vi "DDG64.VI"() -> ()   [LabVIEW 2010]
panel:
  in  "gating":bool
  out "Calculated Kinetic Cycle Time":sgl format="%.2f"
  in  "Frequency (Hz):":dbl format="%.2f"
  in  "Integrate on chip":bool
  in  "Fast insertion delay":bool
  in  "Gate step (nsecs)":i32 step=25
  in  "Pulse Width (nsecs)":i32=1000
  in  "Delay (nsecs)":i32 step=25
  in  "Output A Delay (nsecs)":i32 min=0 step=16
  in  "Gain (0-255)":i32 min=0 max=255
  in  "Kinetic Cycle Time":sgl format="%.2f"
  in  "Shut Down":bool
  in  "Start Acquisition":bool
  out "Graphical Results":i32[](graph)
  out "Return  from Get Acquired Data":u32
  out "Detector X Pixels":i32
  out "Return from GetStatus":u32
  out "Return from Start Acquisition":u32
  in  "Number of Kinetics":i32=5
  out "Return from CheckTimings Exposure":u32
  out "Calculated Exposure Value":sgl format="%.2f"
  in  "Exposure Time (secs)":sgl=0.05 format="%.2f"
  out "Return from Initialize":u32
  in  "Trigger":u32(ring) items=["Internal", "External"]
  # "Status"
  # "Acquisition Mode: Kinetics\nReadout Mode: Full Vertical Binning.  Only showing one track of data."
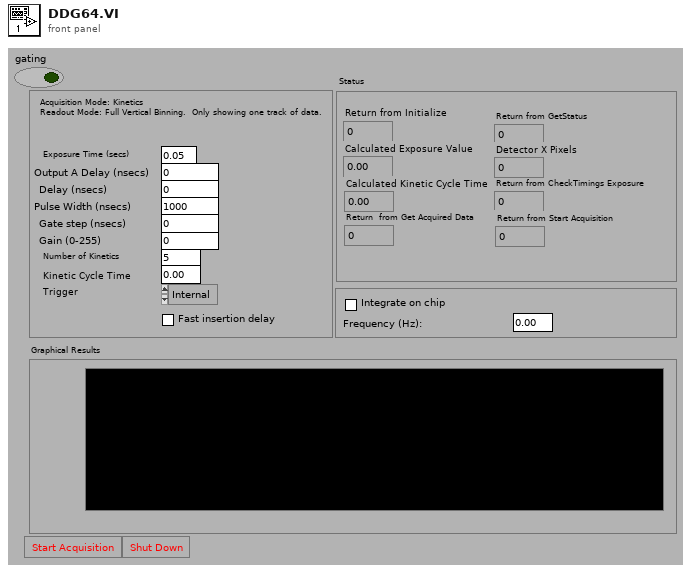
[diagram p1: front panel]
types:
  T1 = typedef "Error Code Enum typedef.ctl" = enum32{"N/A (0)", "DRV_ERROR_CODES", "DRV_SUCCESS", "DRV_VXDNOTINSTALLED", "DRV_ERROR_SCAN", "DRV_ERROR_CHECK_SUM", "DRV_ERROR_FILELOAD", "DRV_UNKNOWN_FUNC", "DRV_ERROR_VXD_INIT", "DRV_ERROR_ADDRESS", "DRV_ERROR_PAGELOCK", "DRV_ERROR_PAGEUNLOCK", "DRV_ERROR_BOARDTEST", "DRV_ERROR_ACK", "DRV_ERROR_UP_FIFO", "DRV_ERROR_PATTERN", "N/A (16)", "DRV_ACQUISITION_ERRORS", "DRV_ACQ_BUFFER", "DRV_ACQ_DOWNFIFO_FULL", "DRV_PROC_UNKONWN_INSTRUCTION", "DRV_ILLEGAL_OP_CODE", "DRV_KINETIC_TIME_NOT_MET", "DRV_ACCUM_TIME_NOT_MET", "DRV_NO_NEW_DATA", "N/A (25)", "DRV_SPOOLERROR", "N/A (27)", "N/A (28)", "N/A (29)", "N/A (30)", "N/A (31)", "N/A (32)", "DRV_TEMPERATURE_CODES", "DRV_TEMPERATURE_OFF", "DRV_TEMPERATURE_NOT_STABILIZED", "DRV_TEMPERATURE_STABILIZED", "DRV_TEMPERATURE_NOT_REACHED", "DRV_TEMPERATURE_OUT_RANGE", "DRV_TEMPERATURE_NOT_SUPPORTED", "DRV_TEMPERATURE_DRIFT", "N/A (41)", "N/A (42)", "N/A (43)", "N/A (44)", "N/A (45)", "N/A (46)", "N/A (47)", "N/A (48)", "DRV_GENERAL_ERRORS", "DRV_INVALID_AUX", "DRV_COF_NOTLOADED", "DRV_FPGAPROG", "DRV_FLEXERROR", "DRV_GPIBERROR", "N/A (55)", "N/A (56)", "N/A (57)", "N/A (58)", "N/A (59)", "N/A (60)", "N/A (61)", "N/A (62)", "N/A (63)", "DRV_DATATYPE", "DRV_DRIVER_ERRORS", "DRV_P1INVALID", "DRV_P2INVALID", "DRV_P3INVALID", "DRV_P4INVALID", "DRV_INIERROR", "DRV_COFERROR", "DRV_ACQUIRING", "DRV_IDLE", "DRV_TEMPCYCLE", "DRV_NOT_INITIALIZED", "DRV_P5INVALID", "DRV_P6INVALID", "DRV_INVALID_MODE", "DRV_INVALID_FILTER", "DRV_I2CERRORS", "DRV_I2CDEVNOTFOUND", "DRV_I2CTIMEOUT", "DRV_P7INVALID", "N/A (84)", "N/A (85)", "N/A (86)", "N/A (87)", "N/A (88)", "N/A (89)", "DRV_IOCERROR", "DRV_VRMVERSIONERROR"}
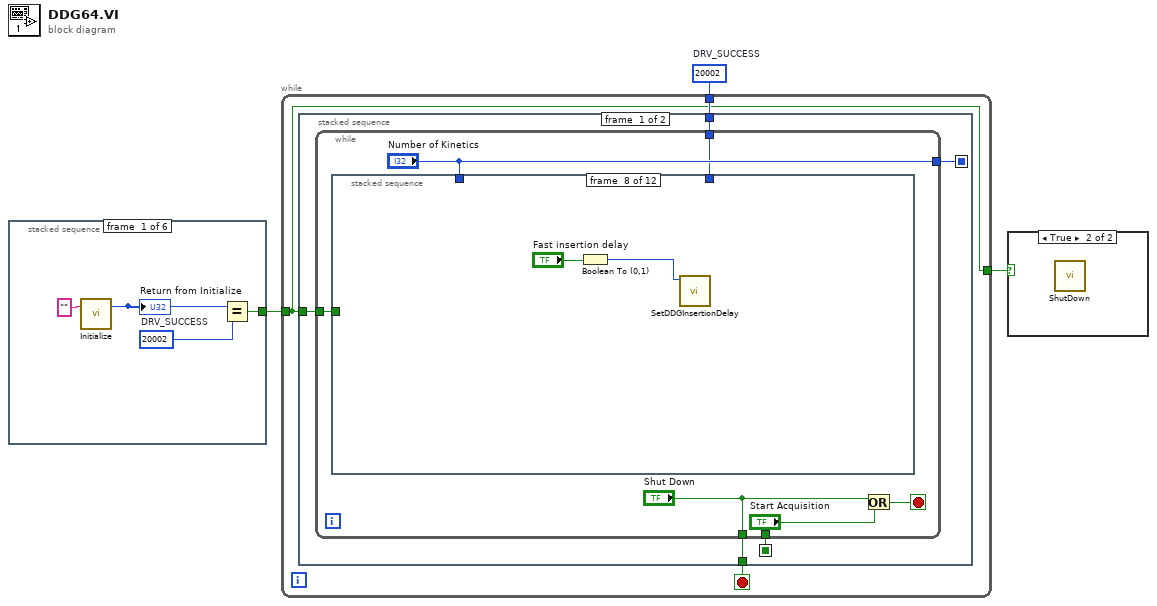
[diagram p0: block diagram]
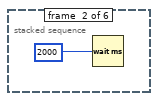
[diagram p2: hidden frame]
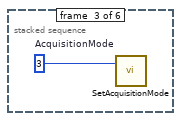
[diagram p3: hidden frame]
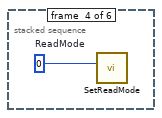
[diagram p4: hidden frame]
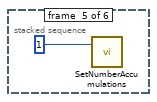
[diagram p5: hidden frame]
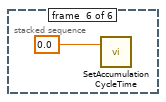
[diagram p6: hidden frame]
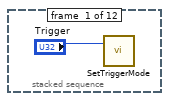
[diagram p8: hidden frame]
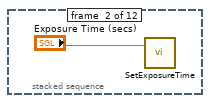
[diagram p9: hidden frame]
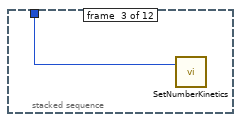
[diagram p10: hidden frame]
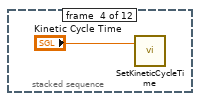
[diagram p11: hidden frame]
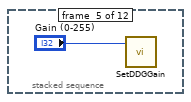
[diagram p12: hidden frame]
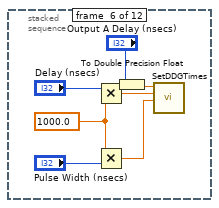
[diagram p13: hidden frame]
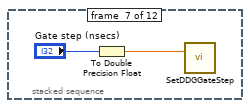
[diagram p14: hidden frame]
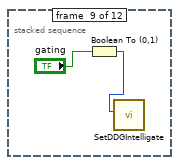
[diagram p15: hidden frame]
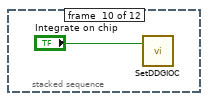
[diagram p16: hidden frame]
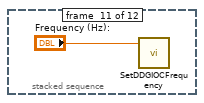
[diagram p17: hidden frame]
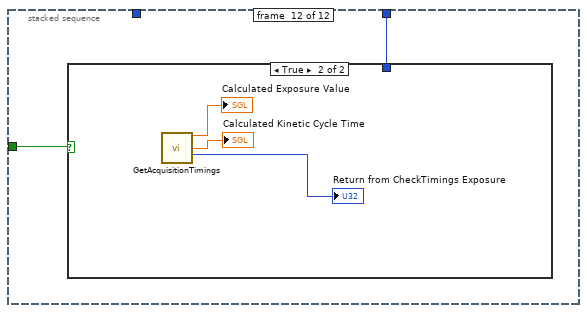
[diagram p18: hidden frame]
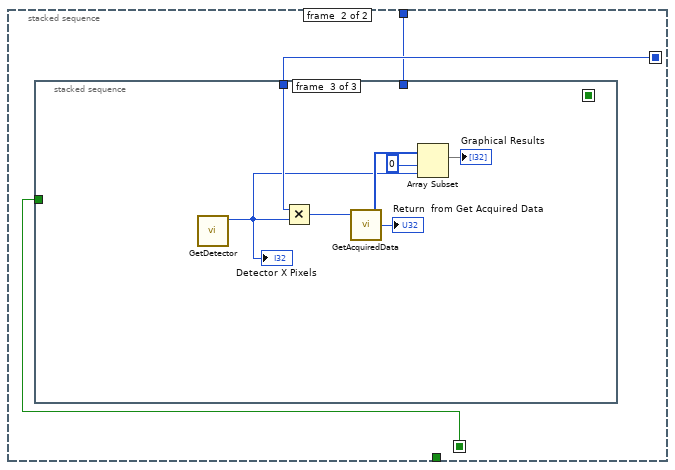
[diagram p20: hidden frame]
diagram:
  w1 = 20002  # DRV_SUCCESS
  n1 = stacked-sequence {
    tunnel: [w4 _ _ _ _ _] -> w2
    frame #0 {
      w5 = 20002  # DRV_SUCCESS
      n2 = call "Initialize.vi"("directory (\"\")"="" ("directory (\"\")")) -> ("DLL error code"=w6:u32)  [unwired: 1 in, 1 out]
      "Return from Initialize" <- w6
      n3 = Equal?(x=w6, y=w5) -> (x = y?=w4:bool)
    }
    frame #1 {
      n4 = Wait (ms)(milliseconds to wait=u32 2000) -> ()  [unwired: 1 out]
    }
    frame #2 {
      w9 = u16 3  # AcquisitionMode
      n5 = call "SetAcquisitionMode.vi"("mode"=w9) -> ()  [unwired: 1 in, 2 out]
    }
    frame #3 {
      w10 = u16 0  # ReadMode
      n6 = call "SetReadMode.vi"("mode"=w10) -> ()  [unwired: 1 in, 2 out]
    }
    frame #4 {
      n7 = call "SetNumberAccumulations.vi"("number"=1) -> ()  [unwired: 1 in, 2 out]
    }
    frame #5 {
      n8 = call "SetAccumulationCycleTime.vi"("time"=sgl 0.0) -> ()  [unwired: 1 in, 2 out]
    }
  }
  n9 = while {
    tunnel: [w13] -> w3
    tunnel: w2 -> [w13]
    tunnel: w1 -> [w14]
    stop <- w15 stop-if-true
    n10 = stacked-sequence {
      seq-local: [w19 _] -> [_ w54]
      seq-local: [w16 _] -> [_ w52]
      tunnel: [w20 _] -> w15
      tunnel: w13 -> [w18 _]
      tunnel: w14 -> [w17 w53]
      frame #0 {
        n11 = while {
          tunnel: ["Shut Down"] -> w20
          tunnel: ["Number of Kinetics"] -> w19
          tunnel: w18 -> [w23]
          tunnel: w17 -> [w22]
          tunnel: ["Start Acquisition"] -> w16
          stop <- w26 stop-if-true
          n12 = stacked-sequence {
            tunnel: "Number of Kinetics" -> [_ _ w29 _ _ _ _ _ _ _ _ _]
            tunnel: w23 -> [_ _ _ _ _ _ _ _ _ _ _ w48]
            tunnel: w22 -> [_ _ _ _ _ _ _ _ _ _ _ w47]
            frame #0 {
              n13 = call "SetTriggerMode.vi"("mode"="Trigger") -> ()  [unwired: 1 in, 2 out]
            }
            frame #1 {
              n14 = call "SetExposureTime.vi"("time"="Exposure Time (secs)") -> ()  [unwired: 1 in, 2 out]
            }
            frame #2 {
              n15 = call "SetNumberKinetics.vi"("number"=w29) -> ()  [unwired: 1 in, 2 out]
            }
            frame #3 {
              n16 = call "SetKineticCycleTime.vi"("time"="Kinetic Cycle Time") -> ()  [unwired: 1 in, 2 out]
            }
            frame #4 {
              n17 = call "SetDDGGain.vi"("gain"="Gain (0-255)") -> ()  [unwired: 1 in, 2 out]
            }
            frame #5 {
              w34 = 1000.0
              n18 = Multiply(x="Delay (nsecs)", y=w34) -> (x*y=w32:dbl)
              n19 = Multiply(x=w34, y="Pulse Width (nsecs)") -> (x*y=w33:dbl)
              n20 = To Double Precision Float(number="Output A Delay (nsecs)") -> (double precision float=w37:dbl)
              n21 = call "SetDDGTimes.vi"("T2"=w33, "T1"=w32, "T0"=w37) -> ()  [unwired: 3 in, 2 out]
            }
            frame #6 {
              n22 = To Double Precision Float(number="Gate step (nsecs)") -> (double precision float=w39:dbl)
              n23 = call "SetDDGGateStep.vi"("step"=w39) -> ()  [unwired: 1 in, 2 out]
            }
            frame #7 {
              n24 = Boolean To (0,1)(Boolean="Fast insertion delay") -> (0, 1=w41:i16)
              n25 = call <userlib>:"SetDDGInsertionDelay.vi"("State"=w41) -> ()  [unwired: 9 in, 2 out]
            }
            frame #8 {
              n26 = Boolean To (0,1)(Boolean="gating") -> (0, 1=w43:i16)
              n27 = call <userlib>:"SetDDGIntelligate.vi"("State"=w43) -> ()  [unwired: 9 in, 2 out]
            }
            frame #9 {
              n28 = call "SetDDGIOC.vi"("integrate"="Integrate on chip") -> ()  [unwired: 1 in, 2 out]
            }
            frame #10 {
              n29 = call "SetDDGIOCFrequency.vi"("frequency"="Frequency (Hz):") -> ()  [unwired: 1 in, 2 out]
            }
            frame #11 {
              n30 = case shown="True" w48 {
                tunnel: w47 -> [_ _]
                frame False {
                }
                frame True {
                  n31 = call "GetAcquisitionTimings.vi"() -> ("exposure"=→"Calculated Exposure Value":sgl, "kinetic"=→"Calculated Kinetic Cycle Time":sgl, "DLL error code"=→"Return from CheckTimings Exposure":u32)  [unwired: 11 in, 2 out]
                }
              }
            }
          }
          n32 = Or(x="Shut Down", y="Start Acquisition") -> (x .or. y?=w26:bool)
        }
      }
      frame #1 {
        n33 = stacked-sequence {
          seq-local: [w56 _ _] -> [_ w62 _]
          tunnel: w53 -> [w57 _ _]
          tunnel: w52 -> [w55 _ _]
          tunnel: w54 -> [_ _ w72]
          frame #0 {
            n34 = case shown="True" w55 {
              tunnel: [FALSE w61] -> w56
              tunnel: w57 -> [_ w59]
              frame False {
              }
              frame True {
                n35 = call "StartAcquisition.vi"() -> ("DLL error code"=w60:u32)  [unwired: 2 in, 1 out]
                "Return from Start Acquisition" <- w60
                n36 = Equal?(x=w59, y=w60) -> (x = y?=w61:bool)
              }
            }
          }
          frame #1 {
            n37 = case shown="True" w62 {
              frame False {
              }
              frame True {
                n38 = while {
                  stop <- w65 continue-if-true
                  w64 = u16 72  # DRV ACQUIRING
                  n39 = Wait Until Next ms Multiple(millisecond multiple=u32 50) -> ()  [unwired: 1 out]
                  n40 = call "GetStatus.vi"() -> ("status"=w63:T1)  [unwired: 3 in, 2 out]
                  "Return from GetStatus" <- w63
                  n41 = Equal?(x=w63, y=w64) -> (x = y?=w65:bool)
                }
              }
            }
          }
          frame #2 {
            n42 = call "GetDetector.vi"() -> ("xpixels"=w68:i32)  [unwired: 4 in, 3 out]
            "Detector X Pixels" <- w68
            n43 = Multiply(x=w72, y=w68) -> (x*y=w71:i32)
            n44 = call "GetAcquiredData.vi"("size"=w71) -> ("DLL error code"=→"Return  from Get Acquired Data":u32, "array"=w69:i32[])  [unwired: 2 in, 1 out]
            n45 = Array Subset(array=w69, index=0, length=w68) -> (→"Graphical Results":i32[])
          }
        }
      }
    }
  }
  n46 = case shown="True" w3 {
    frame False {
    }
    frame True {
      n47 = call "ShutDown.vi"() -> ()  [unwired: 2 in, 2 out]
    }
  }
